vi "createSetTemporaryAddressFrame.vi"(8 "error in (no error)":errorcluster, 9 "TriggerIRQ":bool, 10 "WaitForTrigger":bool, 11 "ILC in":refnum<class "ILC.lvclass">) -> (0 "error out":errorcluster, 2 "Frame":T1 {"Data" format="%02x"}, 3 "ILC out":refnum<class "ILC.lvclass">)   [LabVIEW 2015, in "RTILC.lvlib" / "ILC.lvclass"]
uses:
  ILC.lvclass
  Common_RT_Modbus/DataTypes/Frame.ctl
  Common_RT_Modbus/DynamicFrameBuilder/DynamicFrameBuilder.lvclass
  ILC.lvclass/ILC.ctl
  Common_RT_Modbus/RTModbus.lvlib
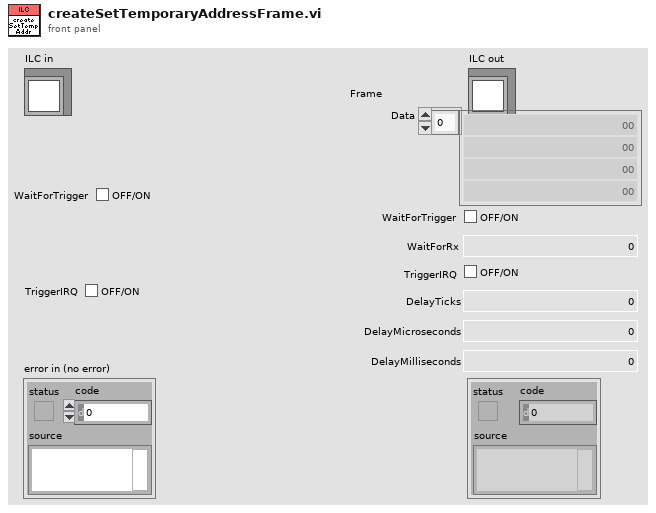
[diagram p1: front panel]
types:
  T1 = typedef "RTModbus.lvlib/Frame.ctl" = cluster{"Data":u8[], "WaitForTrigger":bool, "WaitForRx":u16, "TriggerIRQ":bool, "DelayTicks":u16, "DelayMicroseconds":u16, "DelayMilliseconds":u16}
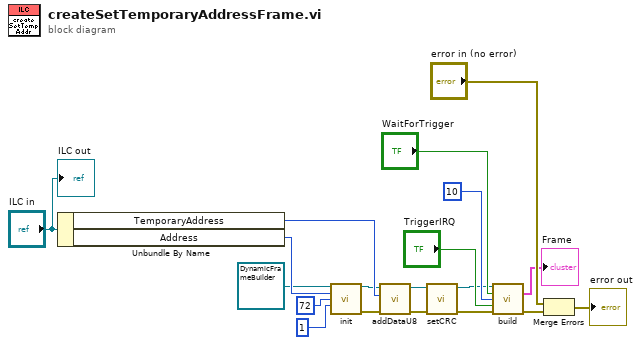
[diagram p0: block diagram]
diagram:
  n1 = Unbundle By Name("ILC in") -> ("TemporaryAddress"=w4:u8, "Address"=w15:u8)
  n2 = call "init.vi"("DynamicFrameBuilder in"=refnum<class "DynamicFrameBuilder.lvclass"> refnum ("RTModbus.lvlib:DynamicFrameBuilder.lvclass"), "Address"=w15, "Function"=u8 72, "DataSize"=1) -> ("DynamicFrameBuilder out"=w3:refnum<class "DynamicFrameBuilder.lvclass">, "error out"=w5:errorcluster)  [unwired: 10 in]
  n3 = call "addDataU8.vi"("error in (no error)"=w5, "Data"=w4, "DynamicFrameBuilder in"=w3) -> ("error out"=w1:errorcluster, "DynamicFrameBuilder out"=w2:refnum<class "DynamicFrameBuilder.lvclass">)  [unwired: 7 in]
  n4 = call "setCRC.vi"("error in (no error)"=w1, "DynamicFrameBuilder in"=w2) -> ("error out"=w13:errorcluster, "DynamicFrameBuilder out"=w7:refnum<class "DynamicFrameBuilder.lvclass">)  [unwired: 8 in]
  n5 = call "build.vi"("DynamicFrameBuilder in"=w7, "WaitForTrigger"="WaitForTrigger", "WaitForRxTimeout"=u16 10, "TriggerIRQ"="TriggerIRQ", "error in (no error)"=w13) -> ("Frame"=→"Frame":T1, "error out"=w8:errorcluster)  [unwired: 8 in, 1 out]
  n6 = Merge Errors("error in (no error)", w8) -> (→"error out":errorcluster)
  "ILC out" <- "ILC in"
